vi "Subscribe to Stopped.vi"(8 "error in (no error)":errorcluster, 11 "API-Reference in":refnum<k1>) -> (0 "error out":errorcluster, 2 "Stopped Event Reg":refnum<event-registration>, 3 "API-Reference out":refnum<k1>)   [LabVIEW 2018, in "Copy of Actor.lvclass"]
uses:
  Copy of Actor.lvclass
  API-Data.ctl
  Stopped.ctl
  Event-References.ctl
  Stop.ctl
  Launched.ctl
  Some Request.ctl
  Some Response.ctl
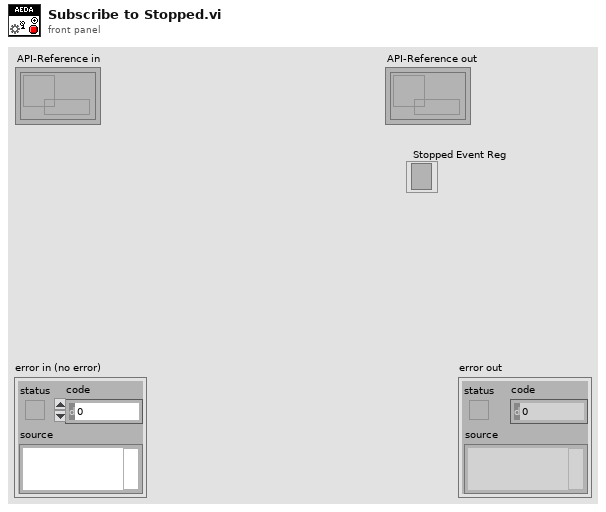
[diagram p1: front panel]
types:
  T1 = typedef "Copy of Actor.lvclass/API-Data.ctl" = cluster{"Launch":refnum<notifier>, "Stopped":refnum<user-event>, "Actor-Events":T2, "Stopped Registration":refnum<event-registration>}
  T2 = typedef "Copy of Actor.lvclass/Event-References.ctl" = cluster{"Stop":refnum<user-event>, "Launched":refnum<user-event>, "Some Request":refnum<user-event>}
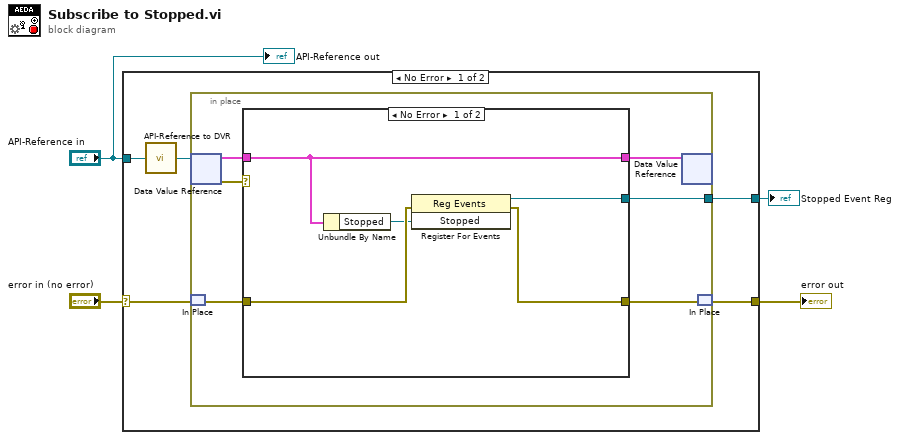
[diagram p0: block diagram]
diagram:
  n1 = case shown="No Error" "error in (no error)" {
    selector: "error in (no error)" -> [w9 w23]
    tunnel: [w8 w23] -> w3
    tunnel: [w7 _] -> w2
    tunnel: "API-Reference in" -> [w5 _]
    frame No Error {
      n2 = call "API-Reference to DVR.vi"("API-Reference in"=w5) -> ("Data Value Reference out"=w6:refnum<data-value>)
      n3 = in-place {
        in-place-border: [w10] -> w7
        n4 = in-place-dvr #1(w6) -> (w14:T1, w15:errorcluster)
        n5 = in-place-match #2(w9) -> (w12:errorcluster)
        n6 = case shown="No Error" w15 {
          selector: w15 -> [_ w22]
          tunnel: w14 -> [w16 w21]
          tunnel: [w16 w21] -> w13
          tunnel: w12 -> [w20 _]
          tunnel: [w19 w22] -> w11
          tunnel: [w18 _] -> w10
          frame No Error {
            n7 = Unbundle By Name(w16) -> ("Stopped"=w17:refnum<user-event>)
            n8 = register-events(error in=w20, w17) -> (reference out=w18:refnum<event-registration>, error out=w19:errorcluster)  [unwired: 1 in]
          }
          frame Error {
          }
        }
        n9 = in-place-dvr #1(w13) -> ()  [unwired: 2 out]
        n10 = in-place-match #2(w11) -> (w8:errorcluster)
      }
    }
    frame Error {
    }
  }
  "error out" <- w3
  "Stopped Event Reg" <- w2
  "API-Reference out" <- "API-Reference in"
